vi "VisionDashRead_BackRight.vi"() -> (0 "BR Ang Deg":dbl, 1 "BR Y Ft":dbl, 2 "BR X Ft":dbl, 3 "BR Error":bool, 4 "BR Time Sec":dbl, 5 "BR Conn":bool, 6 "BR Last Sec Cnt":i64, 7 "BR HasTarg":bool, 8 "BR Count":i64, 11 "BR NewData":bool)   [LabVIEW 2023]
doc: "Vision Network\n\nInput\n --Error in \n\nOutput\n --Error out"
uses:
  <vilib>/Rock Robotics/Network Tables/NT Read Integer.vi
  <vilib>/Rock Robotics/Network Tables/NT Read Boolean.vi
  <vilib>/Rock Robotics/Network Tables/NT Read Number.vi
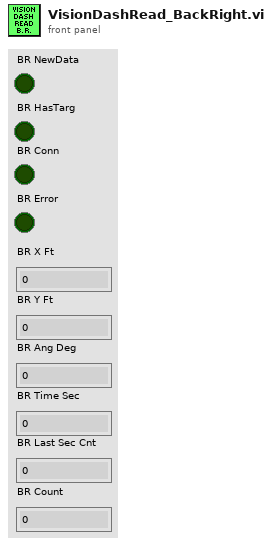
[diagram p1: front panel]
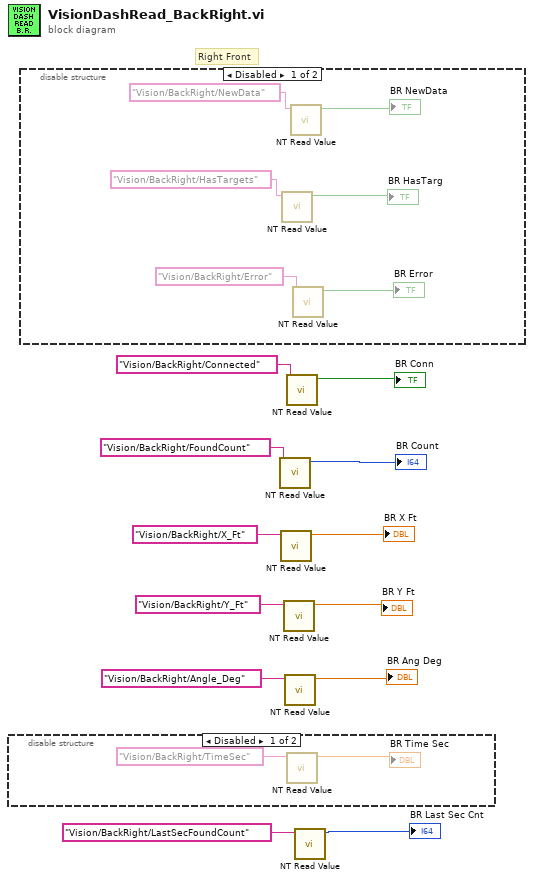
[diagram p0: block diagram]
diagram:
  # "Right Front"
  n1 = disable-structure shown="Disabled" {
    frame Disabled {
      n2 = call-poly <vilib>:"NT Read Value.vi"("name"="Vision/BackRight/TimeSec") -> ("value"=→"BR Time Sec":dbl)  [unwired: 8 in, 2 out]
    }
    frame Enabled {
    }
  }
  n3 = disable-structure shown="Disabled" {
    frame Disabled {
      n4 = call-poly <vilib>:"NT Read Value.vi"("name"="Vision/BackRight/HasTargets") -> ("value"=→"BR HasTarg":bool)  [unwired: 8 in, 2 out]
      n5 = call-poly <vilib>:"NT Read Value.vi"("name"="Vision/BackRight/NewData") -> ("value"=→"BR NewData":bool)  [unwired: 8 in, 2 out]
      n6 = call-poly <vilib>:"NT Read Value.vi"("name"="Vision/BackRight/Error") -> ("value"=→"BR Error":bool)  [unwired: 8 in, 2 out]
    }
    frame Enabled {
    }
  }
  n7 = call-poly <vilib>:"NT Read Value.vi"("name"="Vision/BackRight/FoundCount") -> ("value"=→"BR Count":i64)  [unwired: 8 in, 2 out]
  n8 = call-poly <vilib>:"NT Read Value.vi"("name"="Vision/BackRight/X_Ft") -> ("value"=→"BR X Ft":dbl)  [unwired: 8 in, 2 out]
  n9 = call-poly <vilib>:"NT Read Value.vi"("name"="Vision/BackRight/Y_Ft") -> ("value"=→"BR Y Ft":dbl)  [unwired: 8 in, 2 out]
  n10 = call-poly <vilib>:"NT Read Value.vi"("name"="Vision/BackRight/Angle_Deg") -> ("value"=→"BR Ang Deg":dbl)  [unwired: 8 in, 2 out]
  n11 = call-poly <vilib>:"NT Read Value.vi"("name"="Vision/BackRight/Connected") -> ("value"=→"BR Conn":bool)  [unwired: 8 in, 2 out]
  n12 = call-poly <vilib>:"NT Read Value.vi"("name"="Vision/BackRight/LastSecFoundCount") -> ("value"=→"BR Last Sec Cnt":i64)  [unwired: 8 in, 2 out]
